vi "RT VI.vi"() -> ()   [LabVIEW 2020]
uses:
  <vilib>/FPGAPlugInAG/cRIO-9054/niLvFpga_Open_cRIO-9054.vi
  <vilib>/rvi/interface/common/dynamic/niFpgaDynamicAddResources.vi
  <vilib>/Utility/error.llb/Error Cluster From Error Code.vi
  <vilib>/rvi/errors/niLvFpgaAdjustHostInterfaceError.vi
  <vilib>/FPGAPlugInAG/Dynamic/niLvFpga_Close_Dynamic.vi
  <vilib>/rvi/interface/nirviOpenFPGA/nirviOpenFPGA.xnode
  FPGA Bitfiles/dualpsurtfpgaver_FPGATarget2_fpgaVI_DWnymLJpmZ8.lvbitx
  fpgaVI.vi
  <vilib>/rvi/interface/nirviReadWriteControl/nirviReadWriteControl.xnode
  <vilib>/rvi/interface/nirviCloseFPGA/nirviCloseFPGA.xnode
  <vilib>/rvi/interface/Simulation/niFpgaSimulationCallBeginRW.vi
  NiFpgaLv.dll
panel:
  out "Current Voltage 2":dbl
  in  "Kd 2":dbl
  in  "Ki 2":dbl
  in  "Kp 2":dbl
  in  "EINZEL VOLTAGE 2":dbl(slide) min=0.0 max=500.0 step=0.183 scale=0.0..500.0 scale format="%#_7f"
  in  "Einzel  Enable 2":bool
  out "NI 9264":dbl
  out "NI 9263":dbl
  in  "Einzel  Enable":bool
  in  "ANODE VOLTAGE":dbl(slide) min=0.0 max=500.0 step=0.183 scale=0.0..500.0 scale format="%#_7f"
  in  "Kp":dbl
  in  "Ki":dbl
  in  "Kd":dbl
  out "Current Voltage":dbl
  in  "?":bool
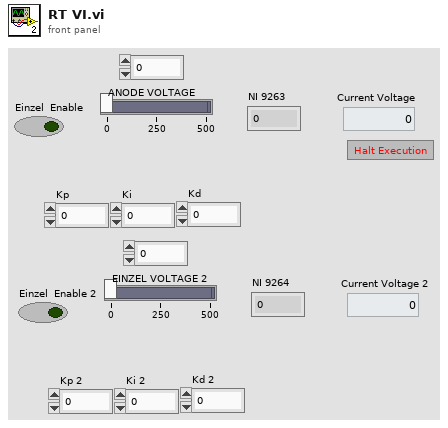
[diagram p1: front panel]
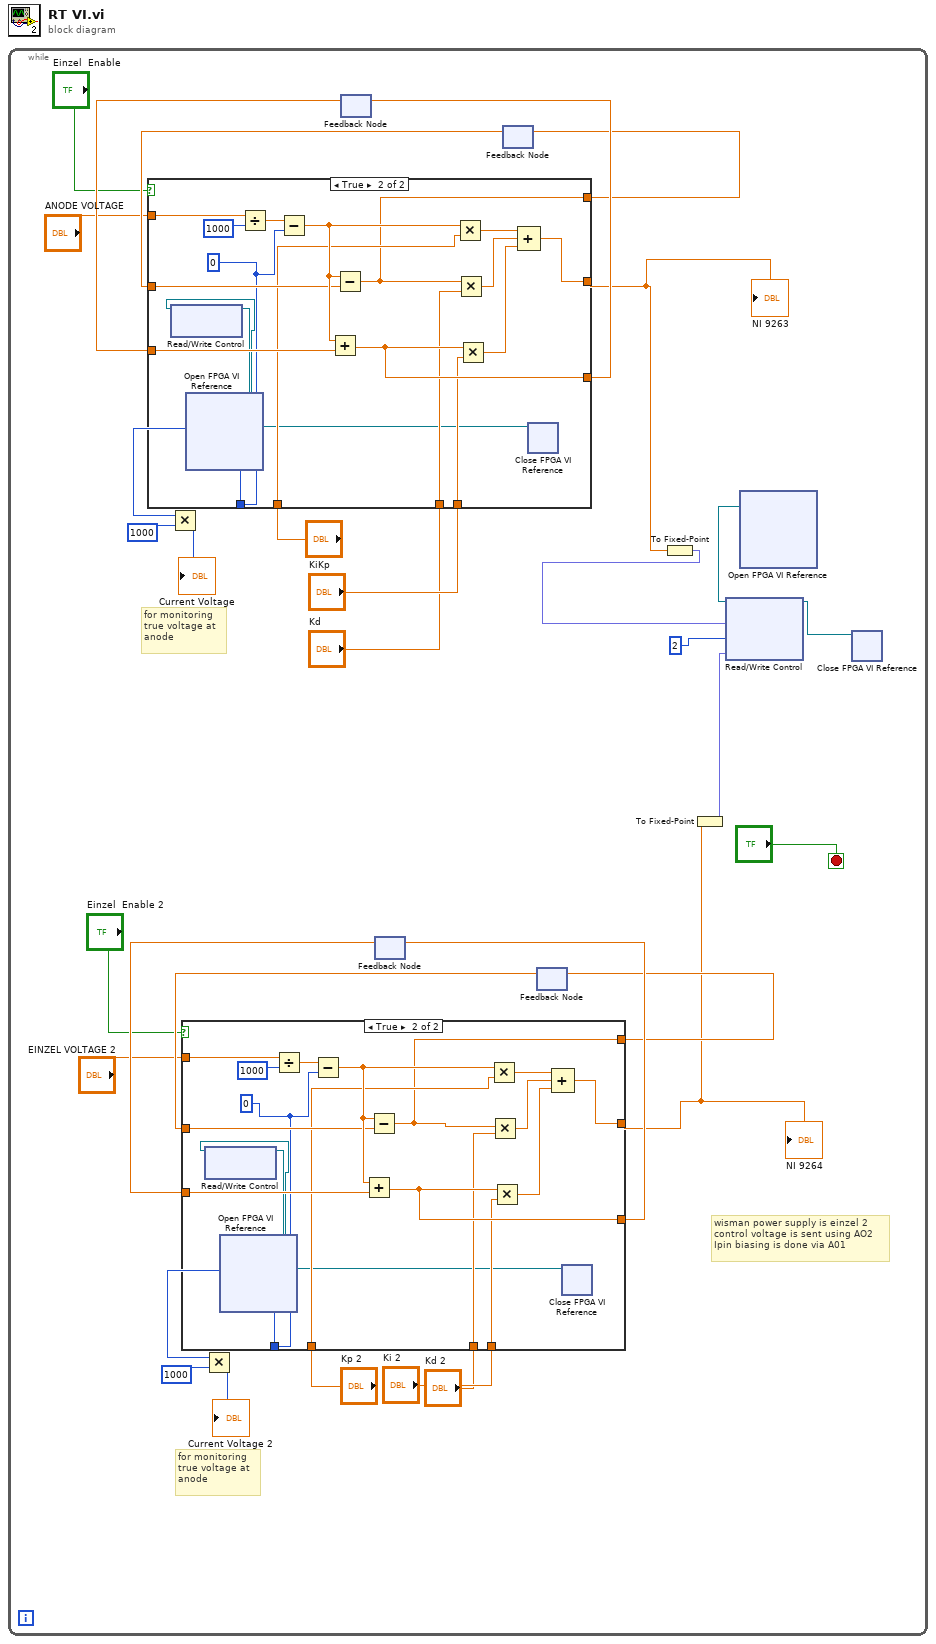
[diagram p0: block diagram]
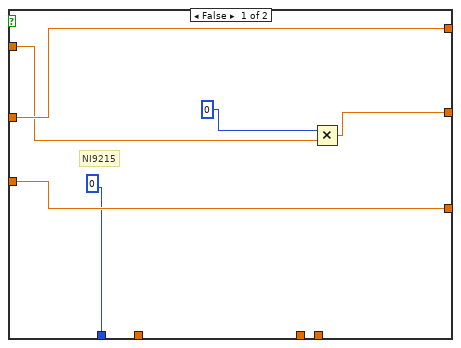
[diagram p2: hidden frame]
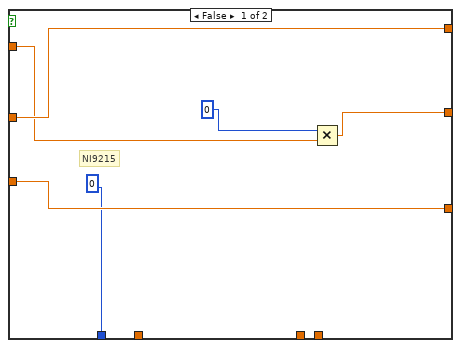
[diagram p3: hidden frame]
diagram:
  n1 = while {
    stop <- "?" stop-if-true
    # "wisman power supply is einzel 2\ncontrol voltage is sent using AO2\nIpin biasing is done via A01"
    # "for monitoring \ntrue voltage at\nanode"
    # "for monitoring \ntrue voltage at\nanode"
    n2 = feedback #1() -> (w31:dbl)  [unwired: 1 in]
    n3 = feedback #2() -> (w15:dbl)  [unwired: 1 in]
    n4 = feedback #3() -> (w32:dbl)  [unwired: 1 in]
    n5 = case shown="True" "Einzel  Enable" {
      tunnel: w32 -> [w62 w74]
      tunnel: [w62 w63] -> w22
      tunnel: w31 -> [w61 w73]
      tunnel: [w61 w72] -> w27
      tunnel: "ANODE VOLTAGE" -> [w59 w71]
      tunnel: [w58 w70] -> w1
      tunnel: "Kp" -> [_ w69]
      tunnel: "Ki" -> [_ w68]
      tunnel: "Kd" -> [_ w67]
      tunnel: [0 w64] -> w23
      frame False {
        # "NI9215"
        n6 = Multiply(x=0, y=w59) -> (x*y=w58:dbl)
      }
      frame True {
        w64 = 0
        n7 = xnode "Open FPGA VI Reference"() -> ("FPGA VI Reference Out"=w65:refnum<k20>)  [unwired: 2 in, 1 out]
        n8 = xnode "Read/Write Control"("FPGA VI Reference In"=w65) -> ("FPGA VI Reference Out"=w66:refnum<k20>)  [unwired: 1 in, 2 out]
        n9 = Divide(x=w71, y=1000) -> (x/y=w76:dbl)
        n10 = Subtract(x=w76, y=w64) -> (x-y=w79:dbl)
        n11 = Add(x=w79, y=w73) -> (x+y=w72:dbl)
        n12 = Subtract(x=w79, y=w74) -> (x-y=w63:dbl)
        n13 = Multiply(x=w79, y=w69) -> (x*y=w77:dbl)
        n14 = Multiply(x=w63, y=w67) -> (x*y=w75:dbl)
        n15 = Multiply(x=w72, y=w68) -> (x*y=w78:dbl)
        n16 = Compound Arithmetic op=ADD(w77, w75, w78) -> (w70:dbl)
        n17 = xnode "Close FPGA VI Reference"("FPGA VI Reference In"=w66) -> ()  [unwired: 1 in, 1 out]
      }
    }
    "NI 9263" <- w1
    n18 = Multiply(x=w23, y=1000) -> (x*y=→"Current Voltage":i32)
    n19 = feedback-in #1(w27) -> ()
    n20 = feedback-in #3(w22) -> ()
    n21 = feedback #4() -> (w16:dbl)  [unwired: 1 in]
    n22 = case shown="True" "Einzel  Enable 2" {
      tunnel: w16 -> [w38 w50]
      tunnel: [w38 w39] -> w6
      tunnel: w15 -> [w37 w49]
      tunnel: [w37 w48] -> w11
      tunnel: "EINZEL VOLTAGE 2" -> [w35 w47]
      tunnel: [w34 w46] -> w4
      tunnel: "Kp 2" -> [_ w45]
      tunnel: "Ki 2" -> [_ w44]
      tunnel: "Kd 2" -> [_ w43]
      tunnel: [0 w40] -> w7
      frame False {
        # "NI9215"
        n23 = Multiply(x=0, y=w35) -> (x*y=w34:dbl)
      }
      frame True {
        w40 = 0
        n24 = xnode "Open FPGA VI Reference"() -> ("FPGA VI Reference Out"=w41:refnum<k20>)  [unwired: 2 in, 1 out]
        n25 = xnode "Read/Write Control"("FPGA VI Reference In"=w41) -> ("FPGA VI Reference Out"=w42:refnum<k20>)  [unwired: 1 in, 2 out]
        n26 = Divide(x=w47, y=1000) -> (x/y=w52:dbl)
        n27 = Subtract(x=w52, y=w40) -> (x-y=w55:dbl)
        n28 = Add(x=w55, y=w49) -> (x+y=w48:dbl)
        n29 = Subtract(x=w55, y=w50) -> (x-y=w39:dbl)
        n30 = Multiply(x=w55, y=w45) -> (x*y=w53:dbl)
        n31 = Multiply(x=w39, y=w43) -> (x*y=w51:dbl)
        n32 = Multiply(x=w48, y=w44) -> (x*y=w54:dbl)
        n33 = Compound Arithmetic op=ADD(w53, w51, w54) -> (w46:dbl)
        n34 = xnode "Close FPGA VI Reference"("FPGA VI Reference In"=w42) -> ()  [unwired: 1 in, 1 out]
      }
    }
    "NI 9264" <- w4
    n35 = Multiply(x=w7, y=1000) -> (x*y=→"Current Voltage 2":i32)
    n36 = feedback-in #2(w11) -> ()
    n37 = feedback-in #4(w6) -> ()
    n38 = To Fixed-Point(number=w1) -> (fixed-point=w19:fxp<+/-,20,5>)  [unwired: 1 in]
    n39 = To Fixed-Point(number=w4) -> (fixed-point=w3:fxp<+/-,20,5>)  [unwired: 1 in]
    n40 = xnode "Open FPGA VI Reference"() -> ("FPGA VI Reference Out"=w17:refnum<k20>)  [unwired: 2 in, 1 out]
    n41 = xnode "Read/Write Control"("FPGA VI Reference In"=w17, "Mod4/AO0"=w19, "Mod4/AO1"=2, "Mod4/AO2"=w3) -> ("FPGA VI Reference Out"=w18:refnum<k20>)  [unwired: 1 in, 1 out]
    n42 = xnode "Close FPGA VI Reference"("FPGA VI Reference In"=w18) -> ()  [unwired: 1 in, 1 out]
  }
